vi "KepcoDCPwr Configure Current Both Protect Levels.vi"(0 "VISA Session":refnum<visa-resource-name>, 5 "Model In":string, 7 "channel name (\"\")":string="\"\"", 11 "error in (no error)":errorcluster {"code" format="%.0x"}, 12 "positive protect":dbl caption="Pos Prot" format="%#.6f", 13 "Neg Prot":dbl format="%#.6f") -> (4 "VISA Session Out":refnum<visa-resource-name>, 6 "Model Out":string, 8 "channel name out (\"\")":string="\"\"" caption="channel name Out (\"\")", 15 "error out":errorcluster {"code" format="%.0x"})   [LabVIEW 2010]
doc: "This VI configures the DC current protect level of a Bi Polar power supply.\n\nThis Vi is not recommended for unipolar Power supplies."
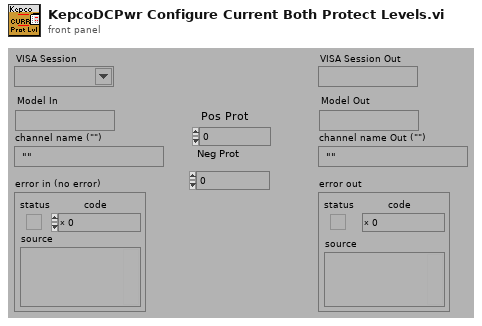
[diagram p1: front panel]
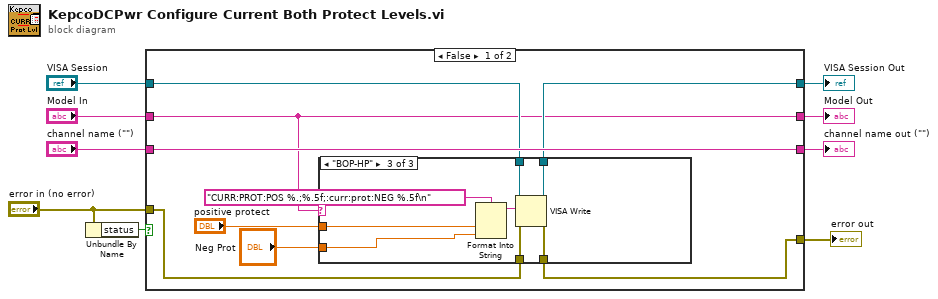
[diagram p0: block diagram]
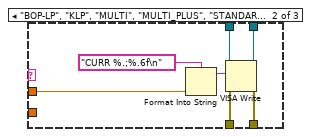
[diagram p3: hidden frame]
diagram:
  n1 = Unbundle By Name("error in (no error)") -> ("status"=w8:bool)
  n2 = case shown="False" w8 {
    tunnel: [w11 w38] -> w9
    tunnel: "error in (no error)" -> [w16 w38]
    tunnel: [w14 w37] -> w6
    tunnel: "VISA Session" -> [w15 w37]
    tunnel: "Model In" -> [w12 w36]
    tunnel: "channel name (\"\")" -> [w17 w35]
    tunnel: [w12 w36] -> w2
    tunnel: [w17 w35] -> w1
    frame False {
      n3 = case shown="\"BOP-HP\"" w12 {
        tunnel: w16 -> [w19 w26 w34]
        tunnel: [w19 w25 w33] -> w11
        tunnel: w15 -> [w18 w24 w32]
        tunnel: [w18 w23 w31] -> w14
        tunnel: "positive protect" -> [_ w22 w30]
        tunnel: "Neg Prot" -> [_ _ w27]
        frame "", Default {
        }
        frame "BOP-LP", "KLP", "MULTI", "MULTI_PLUS", "STANDARD" {
          n4 = Format Into String(format string="CURR %.;%.6f\n", w22) -> (resulting string=w20:string)  [unwired: 2 in, 1 out]
          n5 = VISA Write(VISA resource name=w24, write buffer=w20, error in (no error)=w26) -> (VISA resource name out=w23:refnum<visa-resource-name>, error out=w25:errorcluster)  [unwired: 1 out]
        }
        frame "BOP-HP" {
          n6 = Format Into String(format string="CURR:PROT:POS %.;%.5f;:curr:prot:NEG %.5f\n", w30, w27) -> (resulting string=w28:string)  [unwired: 2 in, 1 out]
          n7 = VISA Write(VISA resource name=w32, write buffer=w28, error in (no error)=w34) -> (VISA resource name out=w31:refnum<visa-resource-name>, error out=w33:errorcluster)  [unwired: 1 out]
        }
      }
    }
    frame True {
    }
  }
  "error out" <- w9
  "VISA Session Out" <- w6
  "channel name out (\"\")" <- w1
  "Model Out" <- w2
